vi "Close.vi"(8 "error in (no error)":errorcluster, 11 "ChromaPowerSupplyModel in":refnum<class "ChromaPowerSupplyModel.lvclass">) -> (0 "error out":errorcluster, 3 "ChromaPowerSupplyModel out":refnum<class "ChromaPowerSupplyModel.lvclass">)   [LabVIEW 2018, in "AcPwrPlugins.lvlib" / "ChromaPowerSupplyModel.lvclass"]
doc: "This VI closes the reference to the instrument(s)."
uses:
  ChromaPowerSupplyModel.lvclass
  ChromaPowerSupplyModel.lvclass/ChromaPowerSupplyModel.ctl
  Database/DatabaseBaseClass/DatabaseBaseClass.lvclass
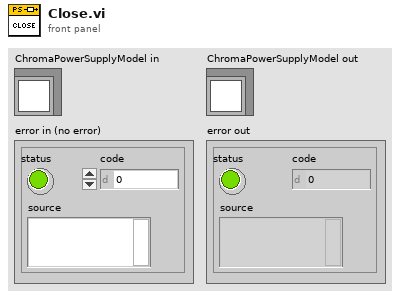
[diagram p1: front panel]
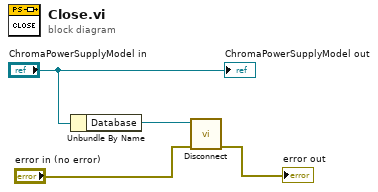
[diagram p0: block diagram]
diagram:
  n1 = Unbundle By Name("ChromaPowerSupplyModel in") -> ("Database"=w4:refnum<class "DatabaseBaseClass.lvclass">)
  n2 = call-dynamic "Disconnect.vi"("error in (no error)"="error in (no error)", "DatabaseBaseClass in"=w4) -> ("error out"=→"error out":errorcluster)  [unwired: 8 in, 1 out]
  "ChromaPowerSupplyModel out" <- "ChromaPowerSupplyModel in"
